vi "Inalfa SCU_LIN Message.vi"(0 "Sequence State in":T2, 1 "LIN Device":T4={"Master Frame(3C)"="MasterReq\nSPA3414_ConfigurationsCMAGeely_CEMCALYPSOSDB34XX0Cfg_LIN3_190709_", "Slave Frame(3D)"="SlaveResp\nSPA3414_ConfigurationsCMAGeely_CEMCALYPSOSDB34XX0Cfg_LIN3_190709_", "Request Schedule"="CEMLIN3DiagRequestSchedule\nSPA3414_ConfigurationsCMAGeely_CEMCALYPSOSDB34XX0Cfg_LIN3_190709_", "Response Schedule"="CEMLIN3DiagResponseSchedule\nSPA3414_ConfigurationsCMAGeely_CEMCALYPSOSDB34XX0Cfg_LIN3_190709_", "Frame Write SCU"="", "Frame Read SCU"="", "LIN Name"=""}, 3 "data bytes log in":string, 4 "Sequence State.Step Description":string, 5 "Sequence State.Step Data String":string, 6 "Mode type":string, 8 "NAD":u8) -> (7 "Software version":string[](array[string]), 10 "Calfile version":string[](array[string]), 11 "Hardware version":string[](array[string]), 12 "data bytes log out":string, 13 "Rx Message":u8[](array[numeric]) format="%02x", 14 "Response Good?":bool, 15 "Error Description":string, 17 "version type":T1(ring), 18 "Sequence State out":T2, 19 "Error No.":u16=132)   [LabVIEW 2018]
uses:
  LIN Device.ctl
  02.Type Def's/sequence state.ctl
  05.UserVI's/sequence/type defs/Sequence Info.ctl
  LIN show messages.ctl
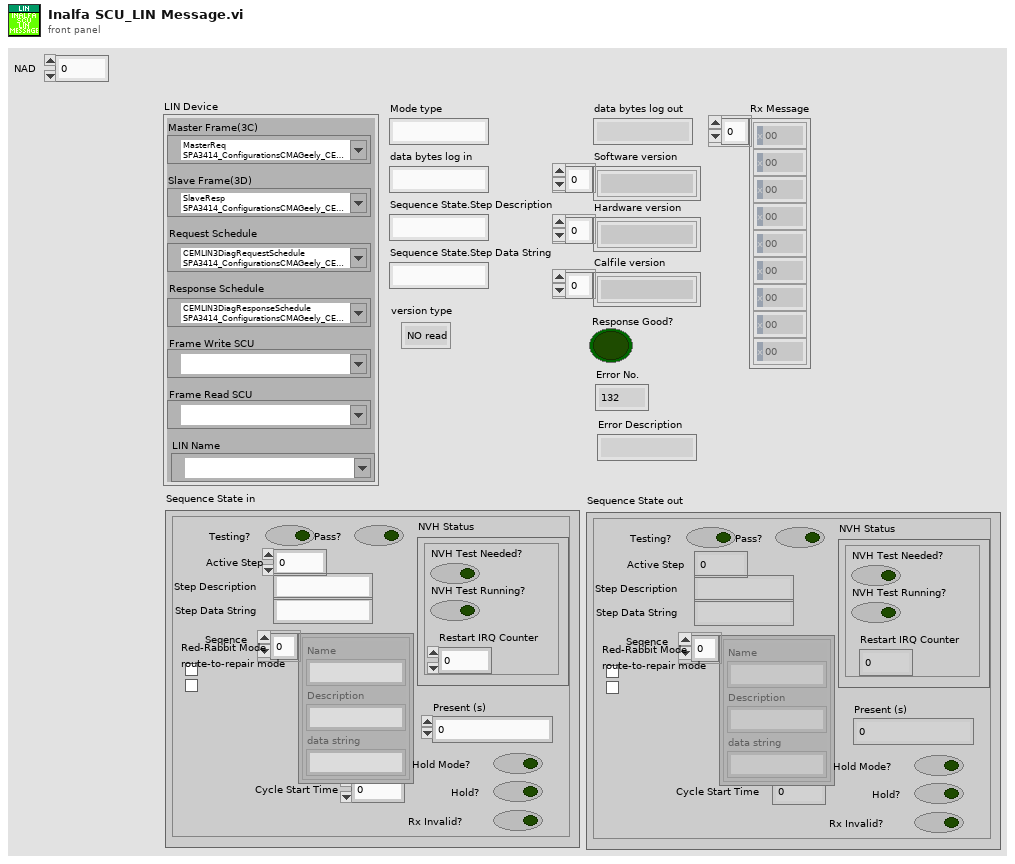
[diagram p1: front panel]
types:
  T1 = enum16{"NO read", "Softeware version", "Hardware version", "Calfile version"}
  T2 = typedef "sequence state.ctl" = cluster{"Step Description":string, "Cycle Start Time":u32, "Step Data String":string, "Pass?":bool, "Seqence":T3[], "Active Step":u8, "Testing?":bool, "Red-Rabbit Mode":bool, "route-to-repair mode":bool, "NVH Status":cluster{"Restart IRQ Counter":u8, "NVH Test Needed?":bool, "NVH Test Running?":bool}, "Present (s)":dbl, "Hold Mode?":bool, "Hold?":bool, "Rx Invalid?":bool}
  T3 = typedef "Sequence Info.ctl" = cluster{"Name":string, "Description":string, "data string":string}
  T4 = typedef "LIN Device.ctl" = cluster{"Master Frame(3C)":refnum<k21>, "Slave Frame(3D)":refnum<k21>, "Request Schedule":refnum<k21>, "Response Schedule":refnum<k21>, "Frame Write SCU":refnum<k21>, "Frame Read SCU":refnum<k21>, "LIN Name":refnum<k21>}
  T5 = typedef "LIN show messages.ctl" = cluster{"Slide Cycles":u16, "Vent Cycles":u16, "String":string, "Tx Bytes":u8[][], "Rx Bytes":u8[], "Only Tx1 Bytes":u8[][], "Go to Position":u16, "Check Glass Position":u16, "Checkgalss":bool, "Check Sunshade Position":u16, "Checksunshade":bool}
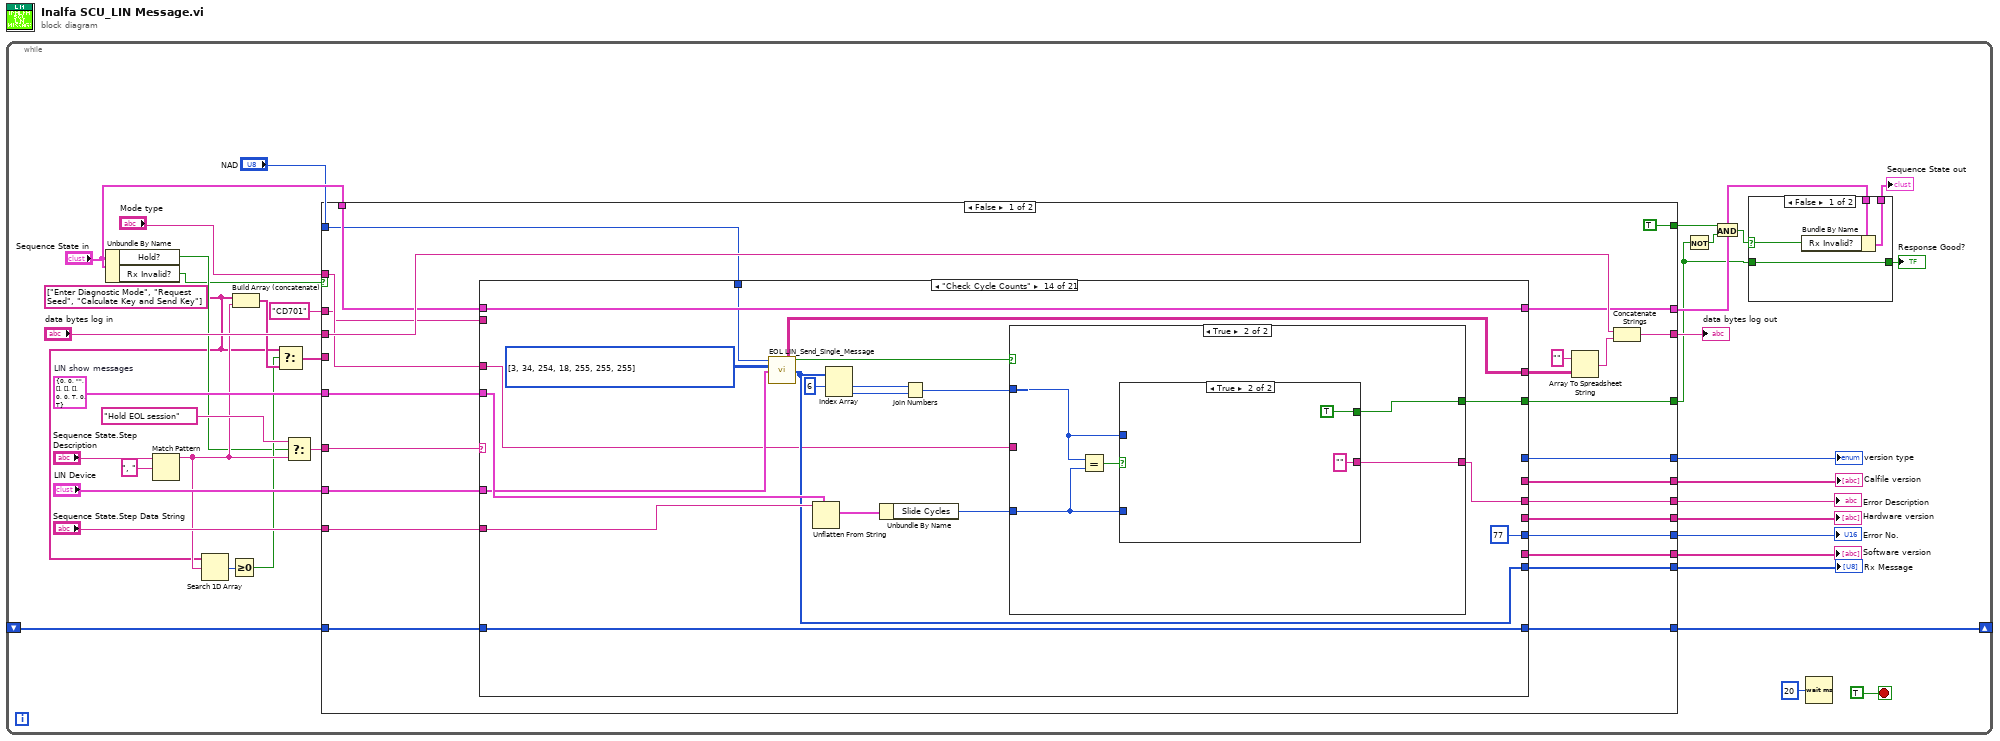
[diagram p0: block diagram]
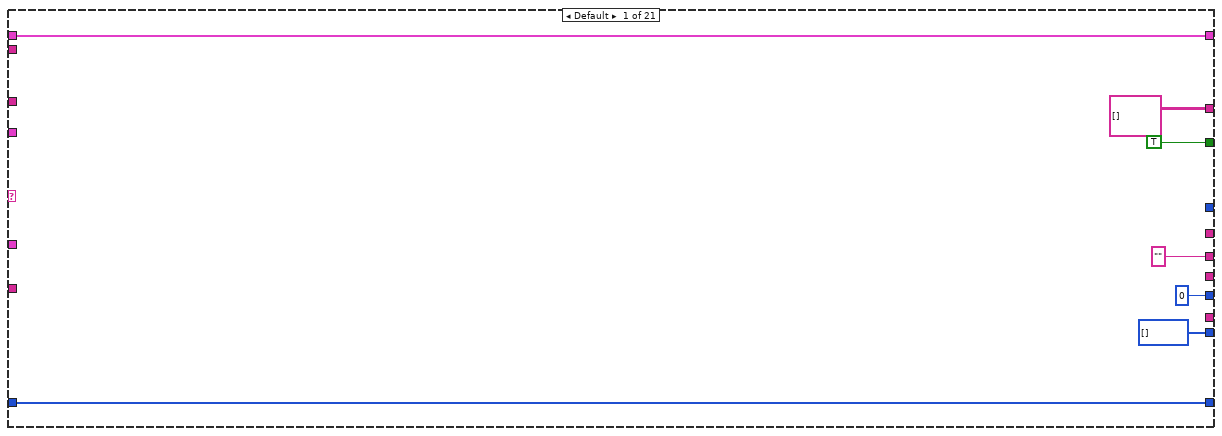
[diagram p2: hidden frame]
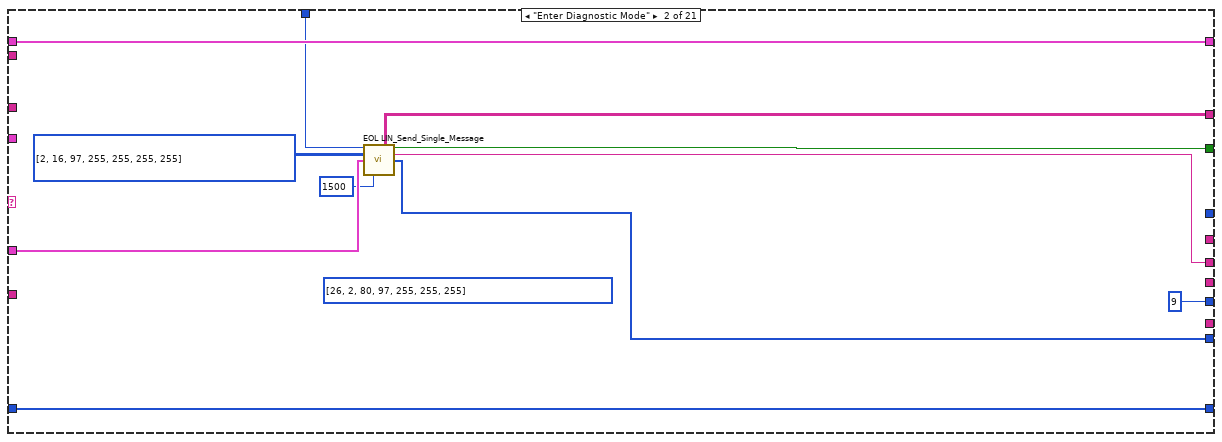
[diagram p3: hidden frame]
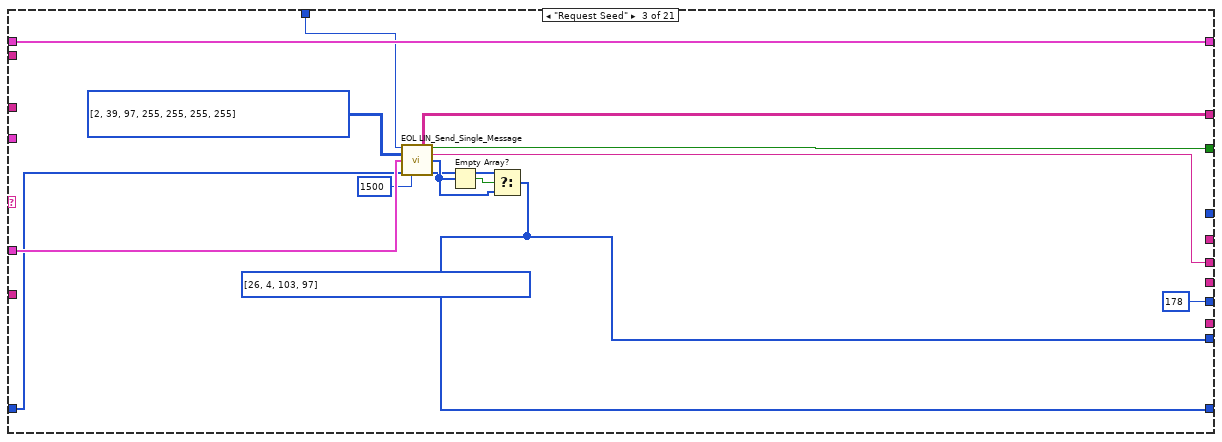
[diagram p4: hidden frame]
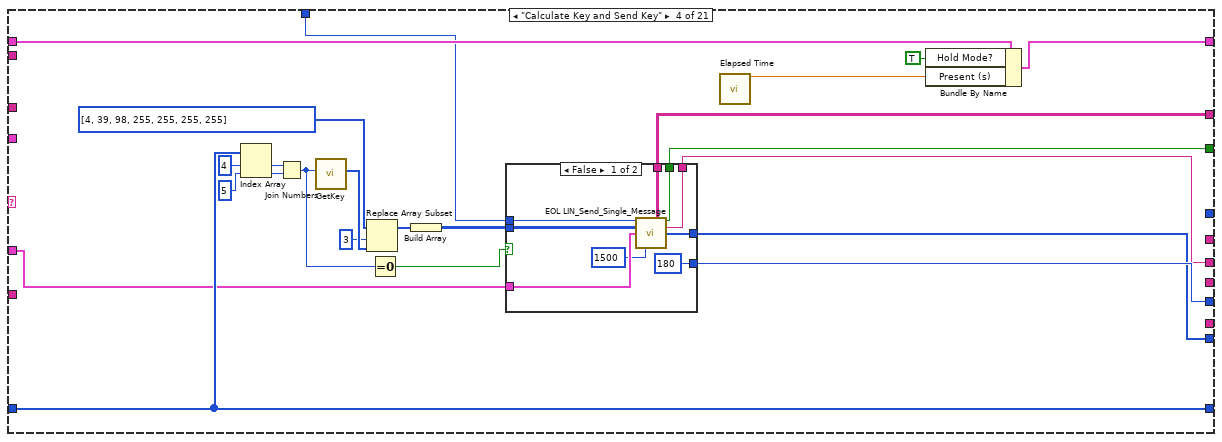
[diagram p5: hidden frame]
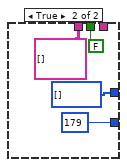
[diagram p6: hidden frame]
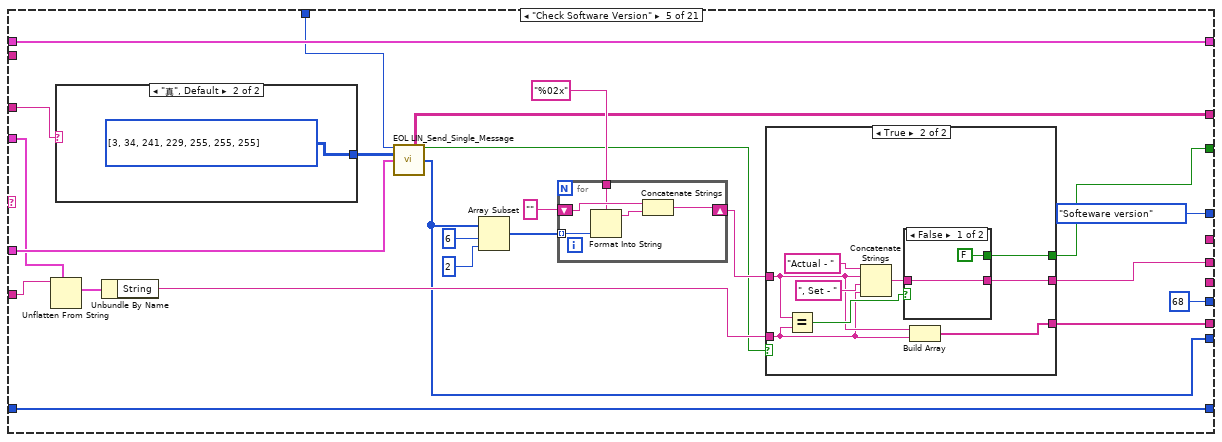
[diagram p7: hidden frame]
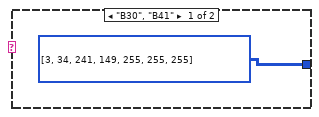
[diagram p8: hidden frame]
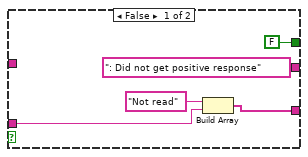
[diagram p9: hidden frame]
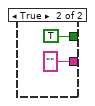
[diagram p10: hidden frame]
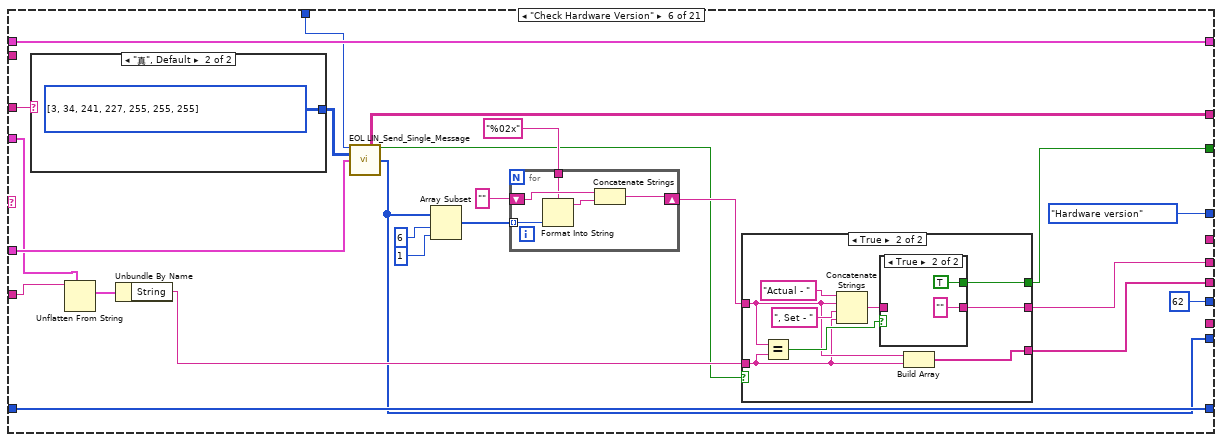
[diagram p11: hidden frame]
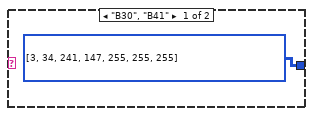
[diagram p12: hidden frame]
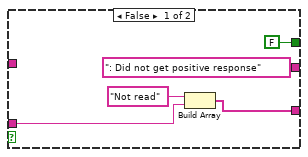
[diagram p13: hidden frame]
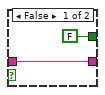
[diagram p14: hidden frame]
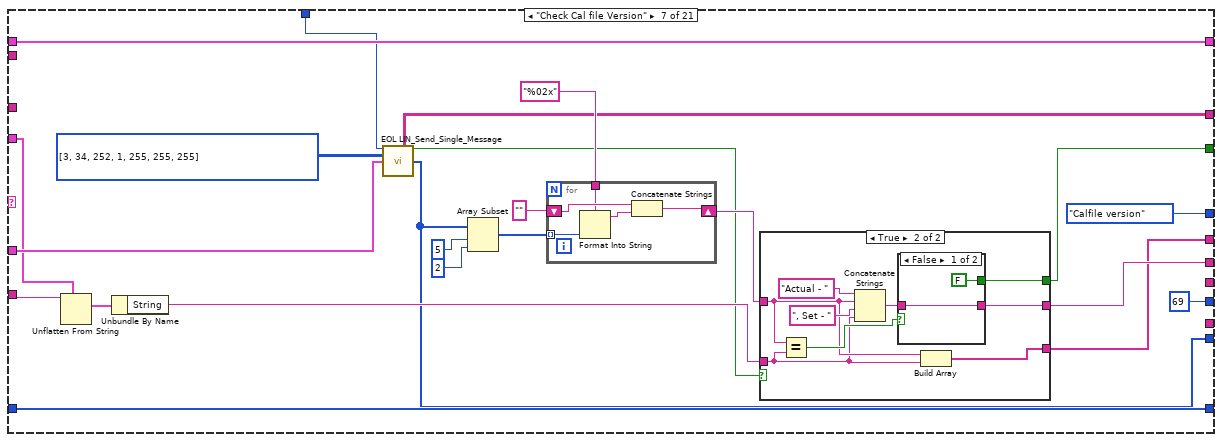
[diagram p15: hidden frame]
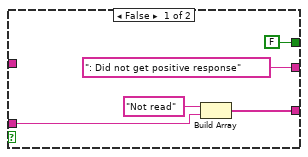
[diagram p16: hidden frame]
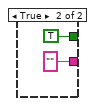
[diagram p17: hidden frame]
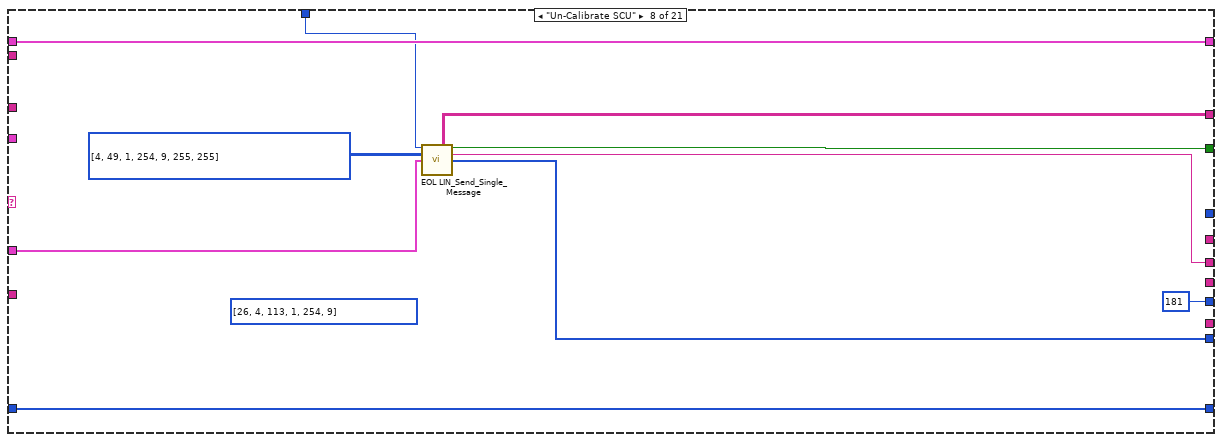
[diagram p18: hidden frame]
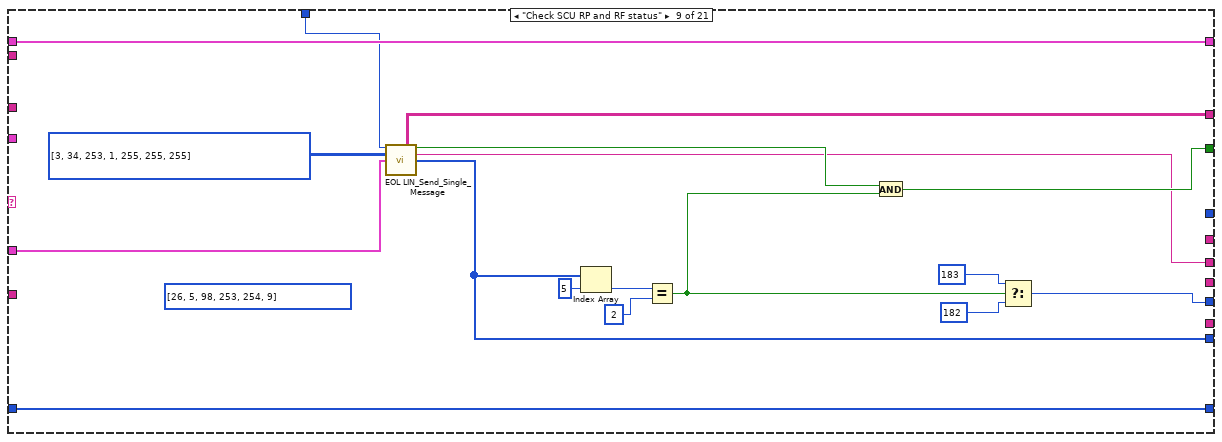
[diagram p19: hidden frame]
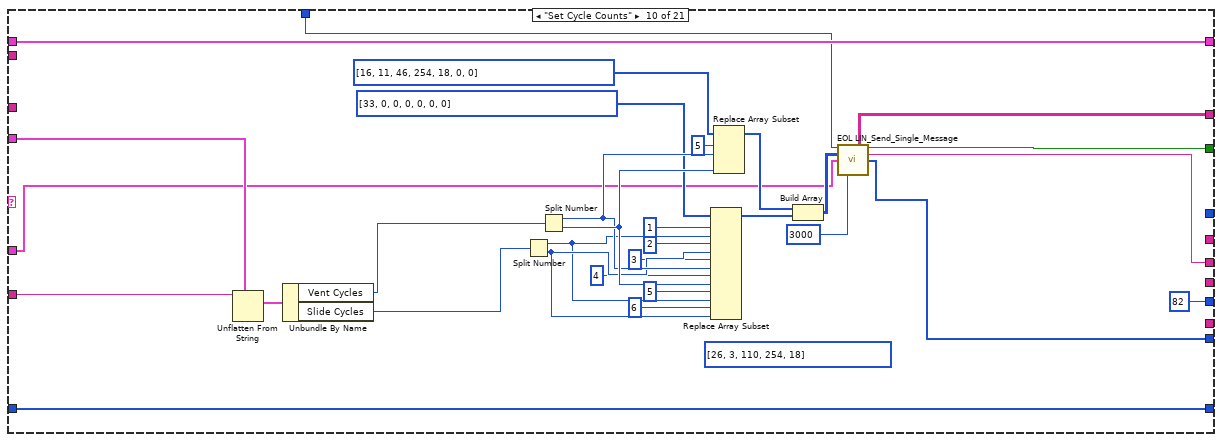
[diagram p20: hidden frame]
diagram:
  n1 = while {
    shift-right: [w33] -> _
    shift-left: _ -> [w32]
    stop <- TRUE stop-if-true
    w11 = string[] ["Enter Diagnostic Mode", "Request Seed", "Calculate Key and Send Key"]
    w36 = T5 {"Slide Cycles"=0, "Vent Cycles"=0, "String"="", "Tx Bytes"=[], "Rx Bytes"=[], "Only Tx1 Bytes"=[], "Go to Position"=0, "Check Glass Position"=0, "Checkgalss"=TRUE, "Check Sunshade Position"=0, "Checksunshade"=TRUE}  # LIN show messages
    n2 = Unbundle By Name("Sequence State in") -> ("Hold?"=w13:bool, "Rx Invalid?"=w12:bool)
    n3 = Match Pattern(string="Sequence State.Step Description", regular expression=", ") -> (before substring=w17:string)  [unwired: 1 in, 3 out]
    n4 = Search 1D Array(1D array=w11, element=w17) -> (index of element=w1:i32)  [unwired: 1 in]
    n5 = Greater Or Equal To 0?(x=w1) -> (x >= 0?=w14:bool)
    n6 = Build Array (concatenate)(w11, w17) -> (w16:string[])
    n7 = Select(t=w11, s=w14, f=w16) -> (s? t:f=w15:string[])
    n8 = Select(t="Hold EOL session", s=w13, f=w17) -> (s? t:f=w30:string)
    n9 = case shown="False" w12 {
      tunnel: "LIN Device" -> [w64 w636]
      tunnel: w36 -> [w63 w637]
      tunnel: [w62 w634] -> w35
      tunnel: [w61 w631] -> w33
      tunnel: w32 -> [w60 w623]
      tunnel: w30 -> [w59 w616]
      tunnel: [w45 w632] -> w20
      tunnel: [w58 w635] -> w3
      tunnel: [w56 w633] -> w26
      tunnel: "Sequence State.Step Data String" -> [w57 w626]
      tunnel: "data bytes log in" -> [w51 w630]
      tunnel: [w53 w629] -> w23
      tunnel: "Sequence State in" -> [w50 w628]
      tunnel: [w49 w627] -> w21
      tunnel: w15 -> [_ w625]
      tunnel: [TRUE FALSE] -> w19
      tunnel: "NAD" -> [w47 w622]
      tunnel: "Mode type" -> [w46 w621]
      tunnel: [w44 w618] -> w9
      tunnel: [w43 w619] -> w8
      tunnel: [w42 w620] -> w7
      tunnel: [w41 w617] -> w6
      tunnel: "CD701" -> [w40 w615]
      frame False {
        n10 = case shown="\"Check Cycle Counts\"" w59 {
          tunnel: w64 -> [_ w81 w92 w103 w154 w194 w245 w284 w301 w309 w343 w364 w394 w493 w528 w538 w546 w559 w576 w587 w610]
          tunnel: [string[][] [] ("TxRx Data") w80 w94 w107 w148 w203 w247 w283 w300 w315 w346 w368 w399 w496 w529 w539 w550 w563 w579 w601 w614] -> w52
          tunnel: [TRUE ("Response Good?") w76 w87 w105 w140 w189 w238 w279 w297 w307 w337 w367 w383 w486 w524 w534 w549 TRUE ("Response Good?") w570 w600 w613] -> w58
          tunnel: w57 -> [_ _ _ _ w146 w195 w243 _ _ w333 w357 w379 w401 w498 _ _ w551 w564 w580 w594 _]
          tunnel: w63 -> [_ _ _ _ w136 w184 w232 _ _ w312 w358 w380 w400 w497 _ _ w552 w565 w581 w595 _]
          tunnel: ["" ("spreadsheet string") w75 w86 w100 w143 w197 w240 w278 w291 w306 w338 w362 w382 w485 w523 w533 w543 w556 w569 w586 w606] -> w62
          tunnel: [u16 0 ("Error No.") u16 9 ("Error No.") u16 178 ("Error No.") w104 u16 68 ("Error No.") u16 62 ("Error No.") u16 69 ("Error No.") u16 181 ("Error No.") w294 u16 82 ("Error No.") u16 184 ("Error No.") u16 185 ("Error No.") u16 20 ("Error No.") u16 77 ("Error No.") u16 55 ("Error No.") u16 55 ("Error No.") u16 56 ("Error No.") u16 0 ("Error No.") u16 56 ("Error No.") u16 186 ("Error No.") u16 187 ("Error No.")] -> w56
          tunnel: [w69 w78 w89 w106 w142 w191 w239 w282 w299 w311 w345 w366 w396 w495 w527 w537 w548 w561 w578 w599 w612] -> w61
          tunnel: w60 -> [w69 w78 w88 w106 w142 w191 w239 w282 w299 w311 w345 w366 w396 w495 w527 w537 w548 w561 w578 w599 w612]
          tunnel: [u8[] [] ("Rx Message") w77 w89 w102 w138 w187 w235 w280 w292 w308 w342 w363 w393 w492 w525 w535 w545 w558 w574 w597 w609] -> w45
          tunnel: w50 -> [w65 w74 w85 w98 w137 w186 w234 w277 w290 w305 w341 w361 w392 w491 w522 w532 w542 w555 w568 w585 w605]
          tunnel: [w65 w74 w85 w97 w137 w186 w234 w277 w290 w305 w341 w361 w392 w491 w522 w532 w542 w555 w568 w585 w604] -> w49
          tunnel: w47 -> [_ w73 w84 w96 w135 w185 w233 w276 w289 w304 w340 w360 w391 w490 w521 w531 w541 w554 w567 w584 w603]
          tunnel: w46 -> [_ _ _ _ w132 w183 _ _ _ _ w336 _ w381 w484 _ _ _ _ _ _ _]
          tunnel: [_ _ _ _ w134 _ _ _ _ _ _ _ _ _ _ _ _ _ _ _ _] -> w44
          tunnel: [_ _ _ _ _ w182 _ _ _ _ _ _ _ _ _ _ _ _ _ _ _] -> w43
          tunnel: [_ _ _ _ _ _ w231 _ _ _ _ _ _ _ _ _ _ _ _ _ _] -> w42
          tunnel: [_ _ _ _ T1."Softeware version" ("version type") T1."Hardware version" ("version type") T1."Calfile version" ("version type") _ _ _ _ _ _ _ _ _ _ _ _ _ _] -> w41
          tunnel: w40 -> [_ _ _ _ _ _ _ _ _ _ w335 _ _ _ _ _ _ _ _ _ _]
          frame Default {
          }
          frame "Enter Diagnostic Mode" {
            (unwired) u8[] [26, 2, 80, 97, 255, 255, 255]
            n11 = call "EOL LIN_Send_Single_Message.vi"("NAD"=w73, "Tx Msg"=u8[][] [[2, 16, 97, 255, 255, 255, 255]], "LIN Device"=w81, "Msg Wait Time"=u32 1500) -> ("TxRx Data"=w80:string[][], "Response Good?"=w76:bool, "spreadsheet string"=w75:string, "Rx Msg"=w77:u8[])  [unwired: 7 in, 1 out]
          }
          frame "Request Seed" {
            (unwired) u8[] [26, 4, 103, 97]
            n12 = call "EOL LIN_Send_Single_Message.vi"("NAD"=w84, "Tx Msg"=u8[][] [[2, 39, 97, 255, 255, 255, 255]], "LIN Device"=w92, "Msg Wait Time"=u32 1500) -> ("TxRx Data"=w94:string[][], "Response Good?"=w87:bool, "spreadsheet string"=w86:string, "Rx Msg"=w90:u8[])  [unwired: 7 in, 1 out]
            n13 = Empty Array?(array=w90) -> (empty?=w91:bool)
            n14 = Select(t=w88, s=w91, f=w90) -> (s? t:f=w89:u8[])
          }
          frame "Calculate Key and Send Key" {
            n15 = Index Array(array=w106, index #1=4 ("index"), index #2=5 ("index")) -> (element #1=w116:u8, element #2=w115:u8)
            n16 = Join Numbers(hi=w116, lo=w115) -> ((hi.lo)=w110:u16)
            n17 = call "GetKey.vi"("x"=w110) -> ("KEY"=w114:u8[])  [unwired: 10 in]
            n18 = Replace Array Subset(array=u8[] [4, 39, 98, 255, 255, 255, 255], new element=w114, index=3) -> (w111:u8[])
            n19 = Equal To 0?(x=w110) -> (x = 0?=w108:bool)
            n20 = Build Array(w111) -> (w109:u8[][])
            n21 = case shown="False" w108 {
              tunnel: w109 -> [w127 _]
              tunnel: [w126 string[][] [] ("TxRx Data")] -> w107
              tunnel: [w125 FALSE ("Response Good?")] -> w105
              tunnel: [w124 _] -> w100
              tunnel: [u16 180 ("Error No.") u16 179 ("Error No.")] -> w104
              tunnel: w103 -> [w122 _]
              tunnel: [w121 u8[] [] ("Rx Message")] -> w102
              tunnel: w96 -> [w120 _]
              frame False {
                n22 = call "EOL LIN_Send_Single_Message.vi"("NAD"=w120, "Tx Msg"=w127, "LIN Device"=w122, "Msg Wait Time"=u32 1500) -> ("TxRx Data"=w126:string[][], "Response Good?"=w125:bool, "spreadsheet string"=w124:string, "Rx Msg"=w121:u8[])  [unwired: 7 in, 1 out]
              }
              frame True {
              }
            }
            n23 = call "Elapsed Time"() -> ("Present (s)"=w101:dbl)  [unwired: 12 in, 7 out]
            n24 = Bundle By Name(cluster=w98, "Hold Mode?"=TRUE, "Present (s)"=w101) -> (w97:T2)
          }
          frame "Check Software Version" {
            n25 = Unflatten From String(type=w136, binary string=w146) -> (value=w147:T5)  [unwired: 3 in, 2 out]
            n26 = case shown="\"真\", Default" w132 {
              tunnel: [u8[][] [[3, 34, 241, 149, 255, 255, 255]] u8[][] [[3, 34, 241, 229, 255, 255, 255]]] -> w155
              frame "B30", "B41" {
              }
              frame "真", Default {
              }
            }
            n27 = Unbundle By Name(w147) -> ("String"=w144:string)
            n28 = call "EOL LIN_Send_Single_Message.vi"("NAD"=w135, "Tx Msg"=w155, "LIN Device"=w154) -> ("TxRx Data"=w148:string[][], "Response Good?"=w141:bool, "Rx Msg"=w138:u8[])  [unwired: 8 in, 2 out]
            n29 = Array Subset(array=w138, index=6, length=2) -> (w153:u8[])
            n30 = for {
              tunnel: w153 -> [w176] mode=indexing
              shift-right: [w179] -> w145
              shift-left: "" -> [w178]
              tunnel: "%02x" ("format string") -> [w177]
              n31 = Format Into String(format string=w177, w176) -> (resulting string=w180:string)  [unwired: 2 in, 1 out]
              n32 = Concatenate Strings(w178, w180) -> (w179:string)
            }
            n33 = case shown="True" w141 {
              tunnel: w145 -> [_ w165]
              tunnel: w144 -> [w159 w164]
              tunnel: [FALSE w167] -> w140
              tunnel: [w158 w163] -> w134
              tunnel: [": Did not get positive response" ("Error Description") w166] -> w143
              frame False {
                n34 = Build Array("Not read" ("Constant level"), w159) -> (w158:string[])
              }
              frame True {
                n35 = Equal?(x=w165, y=w164) -> (x = y?=w168:bool)
                n36 = Concatenate Strings("Actual - " ("string"), w165, ", Set - " ("string"), w164) -> (w169:string)
                n37 = case shown="False" w168 {
                  tunnel: w169 -> [w172 _]
                  tunnel: [FALSE TRUE] -> w167
                  tunnel: [w172 ""] -> w166
                  frame False {
                  }
                  frame True {
                  }
                }
                n38 = Build Array(w165, w164) -> (w163:string[])
              }
            }
          }
          frame "Check Hardware Version" {
            n39 = case shown="\"真\", Default" w183 {
              tunnel: [u8[][] [[3, 34, 241, 147, 255, 255, 255]] u8[][] [[3, 34, 241, 227, 255, 255, 255]]] -> w204
              frame "B30", "B41" {
              }
              frame "真", Default {
              }
            }
            n40 = Unflatten From String(type=w184, binary string=w195) -> (value=w196:T5)  [unwired: 3 in, 2 out]
            n41 = Unbundle By Name(w196) -> ("String"=w193:string)
            n42 = call "EOL LIN_Send_Single_Message.vi"("NAD"=w185, "Tx Msg"=w204, "LIN Device"=w194) -> ("TxRx Data"=w203:string[][], "Response Good?"=w190:bool, "Rx Msg"=w187:u8[])  [unwired: 8 in, 2 out]
            n43 = Array Subset(array=w187, index=6, length=1) -> (w202:u8[])
            n44 = for {
              tunnel: w202 -> [w225] mode=indexing
              shift-right: [w228] -> w192
              shift-left: "" -> [w227]
              tunnel: "%02x" ("format string") -> [w226]
              n45 = Format Into String(format string=w226, w225) -> (resulting string=w229:string)  [unwired: 2 in, 1 out]
              n46 = Concatenate Strings(w227, w229) -> (w228:string)
            }
            n47 = case shown="True" w190 {
              tunnel: w192 -> [_ w214]
              tunnel: w193 -> [w208 w213]
              tunnel: [FALSE w216] -> w189
              tunnel: [w207 w212] -> w182
              tunnel: [": Did not get positive response" ("Error Description") w215] -> w197
              frame False {
                n48 = Build Array("Not read" ("Constant level"), w208) -> (w207:string[])
              }
              frame True {
                n49 = Equal?(x=w214, y=w213) -> (x = y?=w217:bool)
                n50 = Concatenate Strings("Actual - " ("string"), w214, ", Set - " ("string"), w213) -> (w218:string)
                n51 = case shown="True" w217 {
                  tunnel: w218 -> [w221 _]
                  tunnel: [FALSE TRUE] -> w216
                  tunnel: [w221 ""] -> w215
                  frame False {
                  }
                  frame True {
                  }
                }
                n52 = Build Array(w214, w213) -> (w212:string[])
              }
            }
          }
          frame "Check Cal file Version" {
            n53 = Unflatten From String(type=w232, binary string=w243) -> (value=w244:T5)  [unwired: 3 in, 2 out]
            n54 = Unbundle By Name(w244) -> ("String"=w242:string)
            n55 = call "EOL LIN_Send_Single_Message.vi"("NAD"=w233, "Tx Msg"=u8[][] [[3, 34, 252, 1, 255, 255, 255]], "LIN Device"=w245) -> ("TxRx Data"=w247:string[][], "Response Good?"=w237:bool, "Rx Msg"=w235:u8[])  [unwired: 8 in, 2 out]
            n56 = Array Subset(array=w235, index=5, length=2) -> (w252:u8[])
            n57 = for {
              tunnel: w252 -> [w271] mode=indexing
              shift-right: [w274] -> w241
              shift-left: "" -> [w273]
              tunnel: "%02x" ("format string") -> [w272]
              n58 = Format Into String(format string=w272, w271) -> (resulting string=w275:string)  [unwired: 2 in, 1 out]
              n59 = Concatenate Strings(w273, w275) -> (w274:string)
            }
            n60 = case shown="True" w237 {
              tunnel: w241 -> [_ w260]
              tunnel: w242 -> [w254 w259]
              tunnel: [FALSE w262] -> w238
              tunnel: [w253 w258] -> w231
              tunnel: [": Did not get positive response" ("Error Description") w261] -> w240
              frame False {
                n61 = Build Array("Not read" ("Constant level"), w254) -> (w253:string[])
              }
              frame True {
                n62 = Equal?(x=w260, y=w259) -> (x = y?=w263:bool)
                n63 = Concatenate Strings("Actual - " ("string"), w260, ", Set - " ("string"), w259) -> (w264:string)
                n64 = case shown="False" w263 {
                  tunnel: w264 -> [w267 _]
                  tunnel: [FALSE TRUE] -> w262
                  tunnel: [w267 ""] -> w261
                  frame False {
                  }
                  frame True {
                  }
                }
                n65 = Build Array(w260, w259) -> (w258:string[])
              }
            }
          }
          frame "Un-Calibrate SCU" {
            (unwired) u8[] [26, 4, 113, 1, 254, 9]
            n66 = call "EOL LIN_Send_Single_Message.vi"("NAD"=w276, "Tx Msg"=u8[][] [[4, 49, 1, 254, 9, 255, 255]], "LIN Device"=w284) -> ("TxRx Data"=w283:string[][], "Response Good?"=w279:bool, "spreadsheet string"=w278:string, "Rx Msg"=w280:u8[])  [unwired: 8 in, 1 out]
          }
          frame "Check SCU RP and RF status" {
            (unwired) u8[] [26, 5, 98, 253, 254, 9]
            n67 = call "EOL LIN_Send_Single_Message.vi"("NAD"=w289, "Tx Msg"=u8[][] [[3, 34, 253, 1, 255, 255, 255]], "LIN Device"=w301) -> ("TxRx Data"=w300:string[][], "Response Good?"=w298:bool, "spreadsheet string"=w291:string, "Rx Msg"=w292:u8[])  [unwired: 8 in, 1 out]
            n68 = Index Array(array=w292, index=5) -> (element=w287:u8)
            n69 = Equal?(x=w287, y=u8 2 ("element")) -> (x = y?=w286:bool)
            n70 = And(x=w298, y=w286) -> (x .and. y?=w297:bool)
            n71 = Select(t=u16 183 ("Error No."), s=w286, f=u16 182 ("Error No.")) -> (s? t:f=w294:u16)
          }
          frame "Set Cycle Counts" {
            (unwired) u8[] [26, 3, 110, 254, 18]
            n72 = Unflatten From String(type=w312, binary string=w333) -> (value=w332:T5)  [unwired: 3 in, 2 out]
            n73 = Unbundle By Name(w332) -> ("Vent Cycles"=w314:u16, "Slide Cycles"=w313:u16)
            n74 = Split Number(x=w313) -> (hi(x)=w326:u8, lo(x)=w327:u8)
            n75 = Split Number(x=w314) -> (hi(x)=w328:u8, lo(x)=w329:u8)
            n76 = Replace Array Subset(array=u8[] [33, 0, 0, 0, 0, 0, 0] ("Frame payloads to queue"), new element #1=w326, index #1=1 ("索引"), new element #2=w327, index #2=2 ("索引"), new element #3=w328, index #3=3 ("索引"), new element #4=w329, index #4=4 ("索引"), new element #5=w326, index #5=5 ("索引"), new element #6=w327, index #6=6 ("索引")) -> (w331:u8[])
            n77 = Replace Array Subset(array=u8[] [16, 11, 46, 254, 18, 0, 0] ("Frame payloads to queue"), new element #1=w328, index #1=5 ("索引"), new element #2=w329) -> (w330:u8[])  [unwired: 1 in]
            n78 = Build Array(w330, w331) -> (w316:u8[][])
            n79 = call "EOL LIN_Send_Single_Message.vi"("NAD"=w304, "Tx Msg"=w316, "LIN Device"=w309, "Msg Wait Time"=u32 3000) -> ("TxRx Data"=w315:string[][], "Response Good?"=w307:bool, "spreadsheet string"=w306:string, "Rx Msg"=w308:u8[])  [unwired: 7 in, 1 out]
          }
          frame "Go to position glass" {
            n80 = Equal?(x=w335, y=w336) -> (x = y?=w334:bool)
            n81 = Unflatten From String(type=w358, binary string=w357) -> (value=w356:T5)  [unwired: 3 in, 2 out]
            n82 = Unbundle By Name(w356) -> ("Go to Position"=w355:u16)
            n83 = Split Number(x=w355) -> (hi(x)=w352:u8, lo(x)=w351:u8)
            n84 = Replace Array Subset(array=u8[] [33, 0, 0, 0, 0, 255, 255], new element #1=w352, index #1=1 ("index"), new element #2=w351, index #2=2 ("index")) -> (w349:u8[])
            n85 = Build Array(u8[] [16, 9, 49, 1, 253, 4, 1], w349) -> (w347:u8[][])
            n86 = call "EOL LIN_Send_Single_Message.vi"("NAD"=w340, "CD701 position"=w334, "Tx Msg"=w347, "LIN Device"=w343, "Msg Wait Time"=u32 3000) -> ("TxRx Data"=w346:string[][], "Response Good?"=w337:bool, "spreadsheet string"=w338:string, "Rx Msg"=w342:u8[])  [unwired: 6 in, 1 out]
          }
          frame "Go to position sunshade" {
            n87 = Unflatten From String(type=w380, binary string=w379) -> (value=w378:T5)  [unwired: 3 in, 2 out]
            n88 = Unbundle By Name(w378) -> ("Go to Position"=w377:u16)
            n89 = Split Number(x=w377) -> (hi(x)=w374:u8, lo(x)=w373:u8)
            n90 = Replace Array Subset(array=u8[] [33, 0, 0, 0, 0, 255, 255], new element #1=w374, index #1=3 ("index"), new element #2=w373, index #2=4 ("index")) -> (w371:u8[])
            n91 = Build Array(u8[] [16, 9, 49, 1, 253, 4, 2], w371) -> (w369:u8[][])
            n92 = call "EOL LIN_Send_Single_Message.vi"("NAD"=w360, "Tx Msg"=w369, "LIN Device"=w364, "Msg Wait Time"=u32 3000) -> ("TxRx Data"=w368:string[][], "Response Good?"=w367:bool, "spreadsheet string"=w362:string, "Rx Msg"=w363:u8[])  [unwired: 7 in, 1 out]
          }
          frame "Check hall position glass and sunshade" {
            n93 = call "EOL LIN_Send_Single_Message.vi"("NAD"=w391, "Tx Msg"=u8[][] [[3, 34, 253, 2, 255, 255, 255]], "LIN Device"=w394) -> ("TxRx Data"=w399:string[][], "Response Good?"=w390:bool, "Rx Msg"=w393:u8[])  [unwired: 8 in, 2 out]
            n94 = Unflatten From String(type=w400, binary string=w401) -> (value=w402:T5)  [unwired: 3 in, 2 out]
            n95 = Index Array(array=w393, index #1=6 ("index"), index #3=8 ("index")) -> (element #1=w405:u8, element #2=w404:u8, element #3=w398:u8, element #4=w397:u8)  [unwired: 2 in]
            n96 = Unbundle By Name(w402) -> ("Check Glass Position"=w387:u16, "Checkgalss"=w386:bool, "Check Sunshade Position"=w385:u16, "Checksunshade"=w384:bool)
            n97 = Join Numbers(hi=w405, lo=w404) -> ((hi.lo)=w389:u16)
            n98 = Join Numbers(hi=w398, lo=w397) -> ((hi.lo)=w388:u16)
            n99 = case shown="True" w390 {
              tunnel: w389 -> [_ w412]
              tunnel: w387 -> [_ w413]
              tunnel: ["Could not get reponse during Check Motor Hall Position" ("Error Description") w414] -> w382
              tunnel: [FALSE w417] -> w383
              tunnel: w386 -> [_ w416]
              tunnel: w384 -> [_ w415]
              tunnel: w388 -> [_ w411]
              tunnel: w385 -> [_ w418]
              tunnel: w381 -> [_ w410]
              frame False {
              }
              frame True {
                n100 = case shown="\"CD701\"" w410 {
                  tunnel: w418 -> [_ w464]
                  tunnel: [w419 w461] -> w417
                  tunnel: w416 -> [w423 w457]
                  tunnel: w415 -> [_ w453]
                  tunnel: [w422 w449] -> w414
                  tunnel: w413 -> [w421 w448]
                  tunnel: w412 -> [w420 w444]
                  tunnel: w411 -> [_ w443]
                  frame "CD701" {
                    n101 = Not Equal To 0?(x=w420) -> (x != 0?=w433:bool)
                    n102 = Add(x=u16 40, y=w421) -> (x+y=w438:u16)
                    n103 = Subtract(x=w421, y=u16 40) -> (x-y=w435:u16)
                    n104 = In Range and Coerce(upper limit=w438, x=w420, lower limit=w435) -> (In Range?=w432:bool)  [unwired: 1 out]
                    n105 = And(x=w433, y=w432) -> (x .and. y?=w431:bool)
                    n106 = Select(t=w431, s=w423, f=TRUE) -> (s? t:f=w419:bool)
                    n107 = Format Into String(initial string=", Max Lt ", w438) -> (resulting string=w437:string)  [unwired: 2 in, 1 out]
                    n108 = Format Into String(initial string=", Min Lt ", w435) -> (resulting string=w436:string)  [unwired: 2 in, 1 out]
                    n109 = Format Into String(initial string="Glass Actual  " ("string"), w420) -> (resulting string=w439:string)  [unwired: 2 in, 1 out]
                    n110 = Concatenate Strings(w439, w437, w436) -> (w434:string)
                    n111 = Select(t=w434, s=w423, f="") -> (s? t:f=w422:string)
                  }
                  frame "NU2", Default {
                    n112 = Not Equal To 0?(x=w444) -> (x != 0?=w447:bool)
                    n113 = Not Equal To 0?(x=w443) -> (x != 0?=w442:bool)
                    n114 = Add(x=u16 40, y=w448) -> (x+y=w479:u16)
                    n115 = Subtract(x=w448, y=u16 40) -> (x-y=w475:u16)
                    n116 = Add(x=u16 20, y=w464) -> (x+y=w468:u16)
                    n117 = Subtract(x=w464, y=u16 20) -> (x-y=w470:u16)
                    n118 = In Range and Coerce(upper limit=w479, x=w444, lower limit=w475) -> (In Range?=w446:bool)  [unwired: 1 out]
                    n119 = In Range and Coerce(upper limit=w468, x=w443, lower limit=w470) -> (In Range?=w441:bool)  [unwired: 1 out]
                    n120 = And(x=w447, y=w446) -> (x .and. y?=w445:bool)
                    n121 = And(x=w442, y=w441) -> (x .and. y?=w440:bool)
                    n122 = Select(t=w445, s=w457, f=TRUE) -> (s? t:f=w463:bool)
                    n123 = Select(t=w440, s=w453, f=TRUE) -> (s? t:f=w462:bool)
                    n124 = And(x=w463, y=w462) -> (x .and. y?=w461:bool)
                    n125 = Format Into String(initial string="Glass Actual  " ("string"), w444) -> (resulting string=w483:string)  [unwired: 2 in, 1 out]
                    n126 = Format Into String(initial string=", Max Lt ", w479) -> (resulting string=w477:string)  [unwired: 2 in, 1 out]
                    n127 = Format Into String(initial string=", Min Lt ", w475) -> (resulting string=w476:string)  [unwired: 2 in, 1 out]
                    n128 = Format Into String(initial string="。Sunshade Actual  " ("string"), w443) -> (resulting string=w460:string)  [unwired: 2 in, 1 out]
                    n129 = Format Into String(initial string=", Max Lt ", w468) -> (resulting string=w459:string)  [unwired: 2 in, 1 out]
                    n130 = Format Into String(initial string=", Min Lt ", w470) -> (resulting string=w458:string)  [unwired: 2 in, 1 out]
                    n131 = Concatenate Strings(w460, w459, w458) -> (w452:string)
                    n132 = Concatenate Strings(w483, w477, w476) -> (w456:string)
                    n133 = Select(t=w456, s=w457, f="") -> (s? t:f=w451:string)
                    n134 = Select(t=w452, s=w453, f="") -> (s? t:f=w450:string)
                    n135 = Concatenate Strings(w451, w450) -> (w449:string)
                  }
                }
              }
            }
          }
          frame "Check Cycle Counts" {
            n136 = call "EOL LIN_Send_Single_Message.vi"("NAD"=w490, "Tx Msg"=u8[][] [[3, 34, 254, 18, 255, 255, 255]], "LIN Device"=w493) -> ("TxRx Data"=w496:string[][], "Response Good?"=w489:bool, "Rx Msg"=w492:u8[])  [unwired: 8 in, 2 out]
            n137 = Unflatten From String(type=w497, binary string=w498) -> (value=w499:T5)  [unwired: 3 in, 2 out]
            n138 = Index Array(array=w492, index #1=6 ("index")) -> (element #1=w501:u8, element #2=w500:u8)  [unwired: 1 in]
            n139 = Unbundle By Name(w499) -> ("Slide Cycles"=w487:u16)
            n140 = Join Numbers(hi=w501, lo=w500) -> ((hi.lo)=w488:u16)
            n141 = case shown="True" w489 {
              tunnel: w488 -> [_ w509]
              tunnel: w487 -> [_ w508]
              tunnel: ["Could not get reponse during Check Cycle Counts" ("Error Description") w510] -> w485
              tunnel: [FALSE w506] -> w486
              tunnel: w484 -> [_ _]
              frame False {
              }
              frame True {
                n142 = Equal?(x=w509, y=w508) -> (x = y?=w507:bool)
                n143 = case shown="True" w507 {
                  tunnel: [w514 ""] -> w510
                  tunnel: w509 -> [w513 _]
                  tunnel: w508 -> [w512 _]
                  tunnel: [FALSE TRUE] -> w506
                  frame False {
                    n144 = Format Into String(initial string=", Set - ", w512) -> (resulting string=w517:string)  [unwired: 2 in, 1 out]
                    n145 = Format Into String(initial string="Slide Cycle Actual - " ("string"), w513) -> (resulting string=w518:string)  [unwired: 2 in, 1 out]
                    n146 = Concatenate Strings(w518, w517) -> (w514:string)
                  }
                  frame True {
                  }
                }
              }
            }
          }
          frame "Clear DTC" {
            (unwired) u8[] [26, 1, 84]
            n147 = call "EOL LIN_Send_Single_Message.vi"("NAD"=w521, "Tx Msg"=u8[][] [[4, 20, 255, 255, 255, 255, 255]], "LIN Device"=w528) -> ("TxRx Data"=w529:string[][], "Response Good?"=w524:bool, "spreadsheet string"=w523:string, "Rx Msg"=w525:u8[])  [unwired: 8 in, 1 out]
          }
          frame "Check DTC" {
            n148 = call "EOL LIN_Send_Single_Message.vi"("NAD"=w531, "Tx Msg"=u8[][] [[3, 34, 254, 42, 255, 255, 255]], "LIN Device"=w538) -> ("TxRx Data"=w539:string[][], "Response Good?"=w534:bool, "spreadsheet string"=w533:string, "Rx Msg"=w535:u8[])  [unwired: 8 in, 1 out]
          }
          frame "Send Single Message" {
            n149 = Unflatten From String(type=w552, binary string=w551) -> (value=w553:T5)  [unwired: 3 in, 2 out]
            n150 = Unbundle By Name(w553) -> ("Only Tx1 Bytes"=w544:u8[][])
            n151 = call "EOL LIN_Send_Single_Message.vi"("NAD"=w541, "Tx Msg"=w544, "LIN Device"=w546) -> ("TxRx Data"=w550:string[][], "Response Good?"=w549:bool, "spreadsheet string"=w543:string, "Rx Msg"=w545:u8[])  [unwired: 8 in, 1 out]
          }
          frame "Send Single Message With Out Rx" {
            n152 = Unflatten From String(type=w565, binary string=w564) -> (value=w566:T5)  [unwired: 3 in, 2 out]
            n153 = Unbundle By Name(w566) -> ("Only Tx1 Bytes"=w557:u8[][])
            n154 = call "EOL LIN_Send_Single_Message.vi"("NAD"=w554, "Tx Msg"=w557, "LIN Device"=w559) -> ("TxRx Data"=w563:string[][], "spreadsheet string"=w556:string, "Rx Msg"=w558:u8[])  [unwired: 8 in, 2 out]
          }
          frame "Send Single Message With Response" {
            n155 = Unflatten From String(type=w581, binary string=w580) -> (value=w582:T5)  [unwired: 3 in, 2 out]
            n156 = Unbundle By Name(w582) -> ("Tx Bytes"=w575:u8[][], "Rx Bytes"=w573:u8[])
            n157 = call "EOL LIN_Send_Single_Message.vi"("NAD"=w567, "Tx Msg"=w575, "LIN Device"=w576) -> ("TxRx Data"=w579:string[][], "Response Good?"=w572:bool, "spreadsheet string"=w569:string, "Rx Msg"=w574:u8[])  [unwired: 8 in, 1 out]
            n158 = call "Check Response Bytes.vi"("Data Bytes"=w573, "Response Bytes"=w574) -> ("Pass?"=w571:bool)  [unwired: 9 in]
            n159 = And(x=w572, y=w571) -> (x .and. y?=w570:bool)
          }
          frame "Inalfa SCU Teach" {
            (unwired) u8[][] [[5, 49, 1, 240, 0, 0, 255]]
            n160 = Unflatten From String(type=w595, binary string=w594) -> (value=w596:T5)  [unwired: 3 in, 2 out]
            n161 = Unbundle By Name(w596) -> ("String"=w590:string)
            n162 = Decimal String To Number(string=w590, default (0L)=u8 0 ("index (row)")) -> (number=w583:u8)  [unwired: 1 in, 1 out]
            n163 = Replace Array Subset(array=u8[][] [[5, 49, 1, 240, 0, 0, 255]], new element=w583, index (row)=0, index (col)=5 ("disabled index (col)")) -> (w588:u8[][])
            n164 = call "EOL LIN_Send_Single_Message.vi"("NAD"=w584, "Tx Msg"=w588, "LIN Device"=w587) -> ("TxRx Data"=w601:string[][], "Response Good?"=w600:bool, "spreadsheet string"=w586:string, "Rx Msg"=w597:u8[])  [unwired: 8 in, 1 out]
          }
          frame "Hold EOL session" {
            (unwired) u8[][] [[3, 2, 62, 0, 255, 255, 255]]
            n165 = call "EOL LIN_Send_Single_Message.vi"("NAD"=w603, "Tx Msg"=u8[][] [[2, 62, 0, 255, 255, 255, 255]], "LIN Device"=w610) -> ("TxRx Data"=w614:string[][], "Response Good?"=w613:bool, "spreadsheet string"=w606:string, "Rx Msg"=w609:u8[])  [unwired: 8 in, 1 out]
            n166 = call "Elapsed Time2"() -> ("Present (s)"=w607:dbl)  [unwired: 12 in, 7 out]
            n167 = Bundle By Name(cluster=w605, "Hold?"=FALSE ("Hold Mode?"), "Present (s)"=w607) -> (w604:T2)
          }
        }
        n168 = Array To Spreadsheet String(array=w52, 3:"" ("format string")) -> (spreadsheet string=w55:string)  [unwired: 1 in]
        n169 = Concatenate Strings(w51, w55) -> (w53:string)
      }
      frame True {
        n170 = for {
          tunnel: w637 -> [w663]
          tunnel: w636 -> [w662]
          tunnel: [w644] -> w635
          tunnel: [w659] -> w634
          tunnel: [w658] -> w633
          tunnel: [w657] -> w632
          shift-right: [w651] -> w629
          shift-left: w630 -> [w650]
          shift-right: [w660] -> w627
          shift-left: w628 -> [w661]
          tunnel: w626 -> [w649]
          tunnel: w625 -> [w648] mode=indexing
          shift-right: [w656] -> w631
          shift-left: w623 -> [w647]
          tunnel: w622 -> [w646]
          tunnel: w621 -> [w645]
          tunnel: [w643] -> w620
          tunnel: [w642] -> w619
          tunnel: [w641] -> w618
          tunnel: [w640] -> w617
          tunnel: w616 -> [w639]
          tunnel: w615 -> [w638]
          stop <- w644 continue-if-true
          n171 = case shown="\"Enter Diagnostic Mode\"" w648 {
            selector: w648 -> [_ _ _ _ _ _ _ _ _ _ _ _ w986 _ _ _ _ _ _ _ _]
            tunnel: w662 -> [_ w681 w692 w705 w759 w800 w850 w889 w906 w915 w949 w970 w995 w1037 w1133 w1143 w1152 w1165 w1182 w1192 w1215]
            tunnel: [string[][] [] ("TxRx Data") w680 w694 w709 w753 w808 w852 w888 w905 w921 w952 w974 w991 w1042 w1134 w1144 w1156 w1169 w1185 w1206 w1219] -> w652
            tunnel: [TRUE ("Response Good?") w675 w686 w707 w745 w795 w843 w883 w902 w912 w942 w973 w989 w1025 w1128 w1138 w1155 TRUE ("Response Good?") w1176 w1205 w1218] -> w644
            tunnel: w649 -> [_ _ _ _ w741 w791 w838 _ _ w910 w946 w966 w996 w1034 _ _ w1147 w1160 w1173 w1190 _]
            tunnel: w663 -> [_ _ _ _ w751 w789 w848 _ _ w918 w963 w985 w994 w1043 _ _ w1157 w1170 w1186 w1199 _]
            tunnel: ["" ("spreadsheet string") w674 w685 w700 w748 w802 w845 w882 w894 w911 w943 w967 w988 w1024 w1127 w1137 w1148 w1161 w1174 w1191 w1209] -> w659
            tunnel: [u16 0 ("Error No.") u16 9 ("Error No.") u16 178 ("Error No.") w706 u16 68 ("Error No.") u16 62 ("Error No.") u16 69 ("Error No.") u16 181 ("Error No.") w899 u16 82 ("Error No.") u16 184 ("Error No.") u16 185 ("Error No.") u16 20 ("Error No.") u16 20 ("Error No.") u16 55 ("Error No.") u16 55 ("Error No.") u16 56 ("Error No.") u16 0 ("Error No.") u16 56 ("Error No.") u16 186 ("Error No.") u16 187 ("Error No.")] -> w658
            tunnel: [w668 w678 w689 w708 w747 w797 w844 w887 w904 w917 w951 w972 w997 w1039 w1132 w1142 w1154 w1167 w1184 w1204 w1217] -> w656
            tunnel: w647 -> [w668 w678 w688 w708 w747 w797 w844 w887 w904 w917 w951 w972 w997 w1039 w1132 w1142 w1154 w1167 w1184 w1204 w1217]
            tunnel: [u8[] [] ("Rx Message") w677 w689 w704 w743 w793 w840 w885 w896 w914 w948 w969 w992 w1036 w1130 w1140 w1151 w1164 w1180 w1202 w1214] -> w657
            tunnel: w661 -> [w665 w676 w687 w703 w742 w792 w839 w884 w895 w913 w947 w968 w990 w1035 w1129 w1139 w1149 w1162 w1175 w1201 w1211]
            tunnel: [w665 w676 w687 w702 w742 w792 w839 w884 w895 w913 w947 w968 w990 w1035 w1129 w1139 w1149 w1162 w1175 w1201 w1210] -> w660
            tunnel: w646 -> [_ w673 w684 w698 w740 w790 w837 w881 w893 w908 w945 w965 w993 w1033 w1126 w1136 w1146 w1159 w1172 w1189 w1208]
            tunnel: w645 -> [_ _ _ w697 w739 w788 _ _ _ _ w941 _ _ w1023 _ _ _ _ _ _ _]
            tunnel: [_ _ _ _ _ _ w836 _ _ _ _ _ _ _ _ _ _ _ _ _ _] -> w643
            tunnel: [_ _ _ _ _ w787 _ _ _ _ _ _ _ _ _ _ _ _ _ _ _] -> w642
            tunnel: [_ _ _ _ w738 _ _ _ _ _ _ _ _ _ _ _ _ _ _ _ _] -> w641
            tunnel: [_ _ _ _ T1."Softeware version" ("version type") T1."Hardware version" ("version type") T1."Calfile version" ("version type") _ _ _ _ _ _ _ _ _ _ _ _ _ _] -> w640
            tunnel: w639 -> [_ _ _ w696 _ _ _ _ _ _ _ _ _ _ _ _ _ _ _ _ _]
            tunnel: w638 -> [_ _ _ _ _ _ _ _ _ _ w940 _ _ _ _ _ _ _ _ _ _]
            frame Default {
            }
            frame "Enter Diagnostic Mode" {
              (unwired) u8[] [26, 2, 80, 97, 255, 255, 255]
              n172 = call "EOL LIN_Send_Single_Message.vi"("NAD"=w673, "Tx Msg"=u8[][] [[2, 16, 97, 255, 255, 255, 255]], "LIN Device"=w681, "Msg Wait Time"=u32 1000, "Retries"=3) -> ("TxRx Data"=w680:string[][], "Response Good?"=w675:bool, "spreadsheet string"=w674:string, "Rx Msg"=w677:u8[])  [unwired: 6 in, 1 out]
            }
            frame "Request Seed" {
              (unwired) u8[] [26, 4, 103, 97]
              n173 = call "EOL LIN_Send_Single_Message.vi"("NAD"=w684, "Tx Msg"=u8[][] [[2, 39, 97, 255, 255, 255, 255]], "LIN Device"=w692, "Msg Wait Time"=u32 1500) -> ("TxRx Data"=w694:string[][], "Response Good?"=w686:bool, "spreadsheet string"=w685:string, "Rx Msg"=w690:u8[])  [unwired: 7 in, 1 out]
              n174 = Empty Array?(array=w690) -> (empty?=w691:bool)
              n175 = Select(t=w688, s=w691, f=w690) -> (s? t:f=w689:u8[])
            }
            frame "Calculate Key and Send Key" {
              n176 = case shown="\"NU2\", Default" w697 {
                tunnel: [u8[] [4, 39, 2, 255, 255, 255, 255] u8[] [4, 39, 98, 255, 255, 255, 255]] -> w714
                frame "假" {
                }
                frame "NU2", Default {
                }
              }
              n177 = Index Array(array=w708, index #1=4 ("index"), index #2=5 ("index")) -> (element #1=w718:u8, element #2=w717:u8)
              n178 = Join Numbers(hi=w718, lo=w717) -> ((hi.lo)=w712:u16)
              n179 = call "GetKey.vi"("x"=w712) -> ("KEY"=w716:u8[])  [unwired: 10 in]
              n180 = Replace Array Subset(array=w714, new element=w716, index=3) -> (w713:u8[])
              n181 = Equal To 0?(x=w712) -> (x = 0?=w710:bool)
              n182 = Build Array(w713) -> (w711:u8[][])
              n183 = case shown="True" w710 {
                tunnel: w711 -> [w731 _]
                tunnel: [w730 string[][] [] ("TxRx Data")] -> w709
                tunnel: [w729 FALSE ("Response Good?")] -> w707
                tunnel: [w728 w732] -> w700
                tunnel: [u16 180 ("Error No.") u16 179 ("Error No.")] -> w706
                tunnel: w705 -> [w726 _]
                tunnel: [w725 u8[] [] ("Rx Message")] -> w704
                tunnel: w698 -> [w724 _]
                tunnel: w696 -> [_ w732]
                frame False {
                  n184 = call "EOL LIN_Send_Single_Message.vi"("NAD"=w724, "Tx Msg"=w731, "LIN Device"=w726, "Msg Wait Time"=u32 1500) -> ("TxRx Data"=w730:string[][], "Response Good?"=w729:bool, "spreadsheet string"=w728:string, "Rx Msg"=w725:u8[])  [unwired: 7 in, 1 out]
                }
                frame True {
                }
              }
              n185 = call "Elapsed Time3"() -> ("Present (s)"=w701:dbl)  [unwired: 12 in, 7 out]
              n186 = Bundle By Name(cluster=w703, "Hold Mode?"=TRUE, "Present (s)"=w701) -> (w702:T2)
            }
            frame "Check Software Version" {
              n187 = Unflatten From String(type=w751, binary string=w741) -> (value=w752:T5)  [unwired: 3 in, 2 out]
              n188 = case shown="\"假\", Default" w739 {
                tunnel: [u8[][] [[3, 34, 241, 229, 255, 255, 255]] u8[][] [[3, 34, 241, 149, 255, 255, 255]]] -> w760
                frame "假", Default {
                }
                frame "B30", "B41" {
                }
              }
              n189 = Unbundle By Name(w752) -> ("String"=w749:string)
              n190 = call "EOL LIN_Send_Single_Message.vi"("NAD"=w740, "Tx Msg"=w760, "LIN Device"=w759) -> ("TxRx Data"=w753:string[][], "Response Good?"=w746:bool, "Rx Msg"=w743:u8[])  [unwired: 8 in, 2 out]
              n191 = Array Subset(array=w743, index=6, length=2) -> (w758:u8[])
              n192 = for {
                tunnel: w758 -> [w781] mode=indexing
                shift-right: [w784] -> w750
                shift-left: "" -> [w783]
                tunnel: "%02x" ("format string") -> [w782]
                n193 = Format Into String(format string=w782, w781) -> (resulting string=w785:string)  [unwired: 2 in, 1 out]
                n194 = Concatenate Strings(w783, w785) -> (w784:string)
              }
              n195 = case shown="False" w746 {
                tunnel: w750 -> [_ w770]
                tunnel: w749 -> [w764 w769]
                tunnel: [FALSE w772] -> w745
                tunnel: [w763 w768] -> w738
                tunnel: [": Did not get positive response" ("Error Description") w771] -> w748
                frame False {
                  n196 = Build Array("Not read" ("Constant level"), w764) -> (w763:string[])
                }
                frame True {
                  n197 = Equal?(x=w770, y=w769) -> (x = y?=w773:bool)
                  n198 = Concatenate Strings("Actual - " ("string"), w770, ", Set - " ("string"), w769) -> (w774:string)
                  n199 = case shown="True" w773 {
                    tunnel: w774 -> [w777 _]
                    tunnel: [FALSE TRUE] -> w772
                    tunnel: [w777 ""] -> w771
                    frame False {
                    }
                    frame True {
                    }
                  }
                  n200 = Build Array(w770, w769) -> (w768:string[])
                }
              }
            }
            frame "Check Hardware Version" {
              n201 = case shown="\"假\", Default" w788 {
                tunnel: [u8[][] [[3, 34, 241, 227, 255, 255, 255]] u8[][] [[3, 34, 241, 147, 255, 255, 255]]] -> w809
                frame "假", Default {
                }
                frame "B30", "B41" {
                }
              }
              n202 = Unflatten From String(type=w789, binary string=w791) -> (value=w801:T5)  [unwired: 3 in, 2 out]
              n203 = Unbundle By Name(w801) -> ("String"=w799:string)
              n204 = call "EOL LIN_Send_Single_Message.vi"("NAD"=w790, "Tx Msg"=w809, "LIN Device"=w800) -> ("TxRx Data"=w808:string[][], "Response Good?"=w796:bool, "Rx Msg"=w793:u8[])  [unwired: 8 in, 2 out]
              n205 = Array Subset(array=w793, index=6, length=1) -> (w807:u8[])
              n206 = for {
                tunnel: w807 -> [w830] mode=indexing
                shift-right: [w833] -> w798
                shift-left: "" -> [w832]
                tunnel: "%02x" ("format string") -> [w831]
                n207 = Format Into String(format string=w831, w830) -> (resulting string=w834:string)  [unwired: 2 in, 1 out]
                n208 = Concatenate Strings(w832, w834) -> (w833:string)
              }
              n209 = case shown="False" w796 {
                tunnel: w798 -> [_ w819]
                tunnel: w799 -> [w813 w818]
                tunnel: [FALSE w821] -> w795
                tunnel: [w812 w817] -> w787
                tunnel: [": Did not get positive response" ("Error Description") w820] -> w802
                frame False {
                  n210 = Build Array("Not read" ("Constant level"), w813) -> (w812:string[])
                }
                frame True {
                  n211 = Equal?(x=w819, y=w818) -> (x = y?=w822:bool)
                  n212 = Concatenate Strings("Actual - " ("string"), w819, ", Set - " ("string"), w818) -> (w823:string)
                  n213 = case shown="True" w822 {
                    tunnel: w823 -> [w826 _]
                    tunnel: [FALSE TRUE] -> w821
                    tunnel: [w826 ""] -> w820
                    frame False {
                    }
                    frame True {
                    }
                  }
                  n214 = Build Array(w819, w818) -> (w817:string[])
                }
              }
            }
            frame "Check Cal file Version" {
              n215 = Unflatten From String(type=w848, binary string=w838) -> (value=w849:T5)  [unwired: 3 in, 2 out]
              n216 = Unbundle By Name(w849) -> ("String"=w847:string)
              n217 = call "EOL LIN_Send_Single_Message.vi"("NAD"=w837, "Tx Msg"=u8[][] [[3, 34, 252, 1, 255, 255, 255]], "LIN Device"=w850) -> ("TxRx Data"=w852:string[][], "Response Good?"=w842:bool, "Rx Msg"=w840:u8[])  [unwired: 8 in, 2 out]
              n218 = Array Subset(array=w840, index=5, length=2) -> (w857:u8[])
              n219 = for {
                tunnel: w857 -> [w876] mode=indexing
                shift-right: [w879] -> w846
                shift-left: "" -> [w878]
                tunnel: "%02x" ("format string") -> [w877]
                n220 = Format Into String(format string=w877, w876) -> (resulting string=w880:string)  [unwired: 2 in, 1 out]
                n221 = Concatenate Strings(w878, w880) -> (w879:string)
              }
              n222 = case shown="False" w842 {
                tunnel: w846 -> [_ w865]
                tunnel: w847 -> [w859 w864]
                tunnel: [FALSE w867] -> w843
                tunnel: [w858 w863] -> w836
                tunnel: [": Did not get positive response" ("Error Description") w866] -> w845
                frame False {
                  n223 = Build Array("Not read" ("Constant level"), w859) -> (w858:string[])
                }
                frame True {
                  n224 = Equal?(x=w865, y=w864) -> (x = y?=w868:bool)
                  n225 = Concatenate Strings("Actual - " ("string"), w865, ", Set - " ("string"), w864) -> (w869:string)
                  n226 = case shown="True" w868 {
                    tunnel: w869 -> [w872 _]
                    tunnel: [FALSE TRUE] -> w867
                    tunnel: [w872 ""] -> w866
                    frame False {
                    }
                    frame True {
                    }
                  }
                  n227 = Build Array(w865, w864) -> (w863:string[])
                }
              }
            }
            frame "Un-Calibrate SCU" {
              (unwired) u8[] [26, 4, 113, 1, 254, 9]
              n228 = call "EOL LIN_Send_Single_Message.vi"("NAD"=w881, "Tx Msg"=u8[][] [[4, 49, 1, 254, 9, 255, 255]], "LIN Device"=w889) -> ("TxRx Data"=w888:string[][], "Response Good?"=w883:bool, "spreadsheet string"=w882:string, "Rx Msg"=w885:u8[])  [unwired: 8 in, 1 out]
            }
            frame "Check SCU RP and RF status" {
              (unwired) u8[] [26, 5, 98, 253, 254, 9]
              n229 = call "EOL LIN_Send_Single_Message.vi"("NAD"=w893, "Tx Msg"=u8[][] [[3, 34, 253, 1, 255, 255, 255]], "LIN Device"=w906) -> ("TxRx Data"=w905:string[][], "Response Good?"=w903:bool, "spreadsheet string"=w894:string, "Rx Msg"=w896:u8[])  [unwired: 8 in, 1 out]
              n230 = Index Array(array=w896, index=5) -> (element=w892:u8)
              n231 = Equal?(x=w892, y=u8 2 ("element")) -> (x = y?=w891:bool)
              n232 = And(x=w903, y=w891) -> (x .and. y?=w902:bool)
              n233 = Select(t=u16 183 ("Error No."), s=w891, f=u16 182 ("Error No.")) -> (s? t:f=w899:u16)
            }
            frame "Set Cycle Counts" {
              (unwired) u8[] [26, 3, 110, 254, 18]
              n234 = Unflatten From String(type=w918, binary string=w910) -> (value=w938:T5)  [unwired: 3 in, 2 out]
              n235 = Unbundle By Name(w938) -> ("Vent Cycles"=w920:u16, "Slide Cycles"=w919:u16)
              n236 = Split Number(x=w919) -> (hi(x)=w932:u8, lo(x)=w933:u8)
              n237 = Split Number(x=w920) -> (hi(x)=w934:u8, lo(x)=w935:u8)
              n238 = Replace Array Subset(array=u8[] [33, 0, 0, 0, 0, 0, 0] ("Frame payloads to queue"), new element #1=w932, index #1=1 ("索引"), new element #2=w933, index #2=2 ("索引"), new element #3=w934, index #3=3 ("索引"), new element #4=w935, index #4=4 ("索引"), new element #5=w932, index #5=5 ("索引"), new element #6=w933, index #6=6 ("索引")) -> (w937:u8[])
              n239 = Replace Array Subset(array=u8[] [16, 11, 46, 254, 18, 0, 0] ("Frame payloads to queue"), new element #1=w934, index #1=5 ("索引"), new element #2=w935) -> (w936:u8[])  [unwired: 1 in]
              n240 = Build Array(w936, w937) -> (w922:u8[][])
              n241 = call "EOL LIN_Send_Single_Message.vi"("NAD"=w908, "Tx Msg"=w922, "LIN Device"=w915, "Msg Wait Time"=u32 3000) -> ("TxRx Data"=w921:string[][], "Response Good?"=w912:bool, "spreadsheet string"=w911:string, "Rx Msg"=w914:u8[])  [unwired: 7 in, 1 out]
            }
            frame "Go to position glass" {
              n242 = Equal?(x=w941, y=w940) -> (x = y?=w939:bool)
              n243 = Unflatten From String(type=w963, binary string=w946) -> (value=w962:T5)  [unwired: 3 in, 2 out]
              n244 = Unbundle By Name(w962) -> ("Go to Position"=w961:u16)
              n245 = Split Number(x=w961) -> (hi(x)=w958:u8, lo(x)=w957:u8)
              n246 = Replace Array Subset(array=u8[] [33, 0, 0, 0, 0, 255, 255], new element #1=w958, index #1=1 ("index"), new element #2=w957, index #2=2 ("index")) -> (w955:u8[])
              n247 = Build Array(u8[] [16, 9, 49, 1, 253, 4, 1], w955) -> (w953:u8[][])
              n248 = call "EOL LIN_Send_Single_Message.vi"("NAD"=w945, "CD701 position"=w939, "Tx Msg"=w953, "LIN Device"=w949, "Msg Wait Time"=u32 3000) -> ("TxRx Data"=w952:string[][], "Response Good?"=w942:bool, "spreadsheet string"=w943:string, "Rx Msg"=w948:u8[])  [unwired: 6 in, 1 out]
            }
            frame "Go to position sunshade" {
              n249 = Unflatten From String(type=w985, binary string=w966) -> (value=w984:T5)  [unwired: 3 in, 2 out]
              n250 = Unbundle By Name(w984) -> ("Go to Position"=w983:u16)
              n251 = Split Number(x=w983) -> (hi(x)=w980:u8, lo(x)=w979:u8)
              n252 = Replace Array Subset(array=u8[] [33, 0, 0, 0, 0, 255, 255], new element #1=w980, index #1=3 ("index"), new element #2=w979, index #2=4 ("index")) -> (w977:u8[])
              n253 = Build Array(u8[] [16, 9, 49, 1, 253, 4, 2], w977) -> (w975:u8[][])
              n254 = call "EOL LIN_Send_Single_Message.vi"("NAD"=w965, "Tx Msg"=w975, "LIN Device"=w970, "Msg Wait Time"=u32 3000) -> ("TxRx Data"=w974:string[][], "Response Good?"=w973:bool, "spreadsheet string"=w967:string, "Rx Msg"=w969:u8[])  [unwired: 7 in, 1 out]
            }
            frame "Check Cycle Counts" {
              n255 = call "EOL LIN_Send_Single_Message.vi"("NAD"=w993, "Tx Msg"=u8[][] [[3, 34, 254, 18, 255, 255, 255]], "LIN Device"=w995) -> ("TxRx Data"=w991:string[][], "Response Good?"=w1002:bool, "Rx Msg"=w992:u8[])  [unwired: 8 in, 2 out]
              n256 = Unflatten From String(type=w994, binary string=w996) -> (value=w1003:T5)  [unwired: 3 in, 2 out]
              n257 = Index Array(array=w992, index #1=6 ("index")) -> (element #1=w1005:u8, element #2=w1004:u8)  [unwired: 1 in]
              n258 = Unbundle By Name(w1003) -> ("Slide Cycles"=w1000:u16)
              n259 = Join Numbers(hi=w1005, lo=w1004) -> ((hi.lo)=w1001:u16)
              n260 = case shown="True" w1002 {
                tunnel: w1001 -> [_ w1011]
                tunnel: w1000 -> [_ w1010]
                tunnel: ["Could not get reponse during Check Motor Hall Position" ("Error Description") w1012] -> w988
                tunnel: [FALSE w1008] -> w989
                tunnel: w986 -> [_ _]
                frame False {
                }
                frame True {
                  n261 = Equal?(x=w1011, y=w1010) -> (x = y?=w1009:bool)
                  n262 = case shown="True" w1009 {
                    tunnel: [w1016 ""] -> w1012
                    tunnel: w1011 -> [w1015 _]
                    tunnel: w1010 -> [w1014 _]
                    tunnel: [FALSE TRUE] -> w1008
                    frame False {
                      n263 = Format Into String(initial string=", Set - ", w1014) -> (resulting string=w1019:string)  [unwired: 2 in, 1 out]
                      n264 = Format Into String(initial string="Slide Cycle Actual - " ("string"), w1015) -> (resulting string=w1020:string)  [unwired: 2 in, 1 out]
                      n265 = Concatenate Strings(w1020, w1019) -> (w1016:string)
                    }
                    frame True {
                    }
                  }
                }
              }
            }
            frame "Check hall position glass and sunshade" {
              n266 = call "EOL LIN_Send_Single_Message.vi"("NAD"=w1033, "Tx Msg"=u8[][] [[3, 34, 253, 2, 255, 255, 255]], "LIN Device"=w1037) -> ("TxRx Data"=w1042:string[][], "Response Good?"=w1032:bool, "Rx Msg"=w1036:u8[])  [unwired: 8 in, 2 out]
              n267 = Unflatten From String(type=w1043, binary string=w1034) -> (value=w1044:T5)  [unwired: 3 in, 2 out]
              n268 = Index Array(array=w1036, index #1=6 ("index"), index #3=8 ("index")) -> (element #1=w1047:u8, element #2=w1046:u8, element #3=w1041:u8, element #4=w1040:u8)  [unwired: 2 in]
              n269 = Unbundle By Name(w1044) -> ("Check Glass Position"=w1029:u16, "Checkgalss"=w1028:bool, "Check Sunshade Position"=w1027:u16, "Checksunshade"=w1026:bool)
              n270 = Join Numbers(hi=w1047, lo=w1046) -> ((hi.lo)=w1031:u16)
              n271 = Join Numbers(hi=w1041, lo=w1040) -> ((hi.lo)=w1030:u16)
              n272 = case shown="True" w1032 {
                tunnel: w1031 -> [_ w1054]
                tunnel: w1029 -> [_ w1055]
                tunnel: ["Could not get reponse during Check Motor Hall Position" ("Error Description") w1056] -> w1024
                tunnel: [FALSE w1059] -> w1025
                tunnel: w1028 -> [_ w1058]
                tunnel: w1026 -> [_ w1057]
                tunnel: w1030 -> [_ w1053]
                tunnel: w1027 -> [_ w1060]
                tunnel: w1023 -> [_ w1052]
                frame False {
                }
                frame True {
                  n273 = case shown="\"CD701\"" w1052 {
                    tunnel: w1060 -> [_ w1106]
                    tunnel: [w1061 w1103] -> w1059
                    tunnel: w1058 -> [w1062 w1099]
                    tunnel: w1057 -> [_ w1095]
                    tunnel: [w1065 w1091] -> w1056
                    tunnel: w1055 -> [w1063 w1090]
                    tunnel: w1054 -> [w1064 w1086]
                    tunnel: w1053 -> [_ w1085]
                    frame "CD701" {
                      # "只检测玻璃"
                      n274 = Not Equal To 0?(x=w1064) -> (x != 0?=w1075:bool)
                      n275 = Add(x=u16 40, y=w1063) -> (x+y=w1080:u16)
                      n276 = Subtract(x=w1063, y=u16 40) -> (x-y=w1077:u16)
                      n277 = In Range and Coerce(upper limit=w1080, x=w1064, lower limit=w1077) -> (In Range?=w1074:bool)  [unwired: 1 out]
                      n278 = And(x=w1075, y=w1074) -> (x .and. y?=w1073:bool)
                      n279 = Select(t=w1073, s=w1062, f=TRUE) -> (s? t:f=w1061:bool)
                      n280 = Format Into String(initial string=", Max Lt ", w1080) -> (resulting string=w1079:string)  [unwired: 2 in, 1 out]
                      n281 = Format Into String(initial string=", Min Lt ", w1077) -> (resulting string=w1078:string)  [unwired: 2 in, 1 out]
                      n282 = Format Into String(initial string="Glass Actual  " ("string"), w1064) -> (resulting string=w1081:string)  [unwired: 2 in, 1 out]
                      n283 = Concatenate Strings(w1081, w1079, w1078) -> (w1076:string)
                      n284 = Select(t=w1076, s=w1062, f="") -> (s? t:f=w1065:string)
                    }
                    frame "NU2", Default {
                      n285 = Not Equal To 0?(x=w1086) -> (x != 0?=w1089:bool)
                      n286 = Not Equal To 0?(x=w1085) -> (x != 0?=w1084:bool)
                      n287 = Add(x=u16 40, y=w1090) -> (x+y=w1121:u16)
                      n288 = Subtract(x=w1090, y=u16 40) -> (x-y=w1117:u16)
                      n289 = Add(x=u16 20, y=w1106) -> (x+y=w1110:u16)
                      n290 = Subtract(x=w1106, y=u16 20) -> (x-y=w1112:u16)
                      n291 = In Range and Coerce(upper limit=w1121, x=w1086, lower limit=w1117) -> (In Range?=w1088:bool)  [unwired: 1 out]
                      n292 = In Range and Coerce(upper limit=w1110, x=w1085, lower limit=w1112) -> (In Range?=w1083:bool)  [unwired: 1 out]
                      n293 = And(x=w1089, y=w1088) -> (x .and. y?=w1087:bool)
                      n294 = And(x=w1084, y=w1083) -> (x .and. y?=w1082:bool)
                      n295 = Select(t=w1087, s=w1099, f=TRUE) -> (s? t:f=w1105:bool)
                      n296 = Select(t=w1082, s=w1095, f=TRUE) -> (s? t:f=w1104:bool)
                      n297 = And(x=w1105, y=w1104) -> (x .and. y?=w1103:bool)
                      n298 = Format Into String(initial string=", Max Lt ", w1121) -> (resulting string=w1119:string)  [unwired: 2 in, 1 out]
                      n299 = Format Into String(initial string=", Min Lt ", w1117) -> (resulting string=w1118:string)  [unwired: 2 in, 1 out]
                      n300 = Format Into String(initial string="。Sunshade Actual  " ("string"), w1085) -> (resulting string=w1102:string)  [unwired: 2 in, 1 out]
                      n301 = Format Into String(initial string=", Max Lt ", w1110) -> (resulting string=w1101:string)  [unwired: 2 in, 1 out]
                      n302 = Format Into String(initial string=", Min Lt ", w1112) -> (resulting string=w1100:string)  [unwired: 2 in, 1 out]
                      n303 = Format Into String(initial string="Glass Actual  " ("string"), w1086) -> (resulting string=w1125:string)  [unwired: 2 in, 1 out]
                      n304 = Concatenate Strings(w1102, w1101, w1100) -> (w1094:string)
                      n305 = Concatenate Strings(w1125, w1119, w1118) -> (w1098:string)
                      n306 = Select(t=w1098, s=w1099, f="") -> (s? t:f=w1093:string)
                      n307 = Select(t=w1094, s=w1095, f="") -> (s? t:f=w1092:string)
                      n308 = Concatenate Strings(w1093, w1092) -> (w1091:string)
                    }
                  }
                }
              }
            }
            frame "Clear DTC" {
              (unwired) u8[] [26, 1, 84]
              n309 = call "EOL LIN_Send_Single_Message.vi"("NAD"=w1126, "Tx Msg"=u8[][] [[4, 20, 255, 255, 255, 255, 255]], "LIN Device"=w1133) -> ("TxRx Data"=w1134:string[][], "Response Good?"=w1128:bool, "spreadsheet string"=w1127:string, "Rx Msg"=w1130:u8[])  [unwired: 8 in, 1 out]
            }
            frame "Check DTC" {
              (unwired) u8[] [26, 1, 84]
              n310 = call "EOL LIN_Send_Single_Message.vi"("NAD"=w1136, "Tx Msg"=u8[][] [[3, 34, 254, 42, 255, 255, 255]], "LIN Device"=w1143) -> ("TxRx Data"=w1144:string[][], "Response Good?"=w1138:bool, "spreadsheet string"=w1137:string, "Rx Msg"=w1140:u8[])  [unwired: 8 in, 1 out]
            }
            frame "Send Single Message" {
              n311 = Unflatten From String(type=w1157, binary string=w1147) -> (value=w1158:T5)  [unwired: 3 in, 2 out]
              n312 = Unbundle By Name(w1158) -> ("Only Tx1 Bytes"=w1150:u8[][])
              n313 = call "EOL LIN_Send_Single_Message.vi"("NAD"=w1146, "Tx Msg"=w1150, "LIN Device"=w1152) -> ("TxRx Data"=w1156:string[][], "Response Good?"=w1155:bool, "spreadsheet string"=w1148:string, "Rx Msg"=w1151:u8[])  [unwired: 8 in, 1 out]
            }
            frame "Send Single Message With Out Rx" {
              n314 = Unflatten From String(type=w1170, binary string=w1160) -> (value=w1171:T5)  [unwired: 3 in, 2 out]
              n315 = Unbundle By Name(w1171) -> ("Only Tx1 Bytes"=w1163:u8[][])
              n316 = call "EOL LIN_Send_Single_Message.vi"("NAD"=w1159, "Tx Msg"=w1163, "LIN Device"=w1165) -> ("TxRx Data"=w1169:string[][], "spreadsheet string"=w1161:string, "Rx Msg"=w1164:u8[])  [unwired: 8 in, 2 out]
            }
            frame "Send Single Message With Response" {
              n317 = Unflatten From String(type=w1186, binary string=w1173) -> (value=w1187:T5)  [unwired: 3 in, 2 out]
              n318 = Unbundle By Name(w1187) -> ("Tx Bytes"=w1181:u8[][], "Rx Bytes"=w1179:u8[])
              n319 = call "EOL LIN_Send_Single_Message.vi"("NAD"=w1172, "Tx Msg"=w1181, "LIN Device"=w1182) -> ("TxRx Data"=w1185:string[][], "Response Good?"=w1178:bool, "spreadsheet string"=w1174:string, "Rx Msg"=w1180:u8[])  [unwired: 8 in, 1 out]
              n320 = call "Check Response Bytes.vi"("Data Bytes"=w1179, "Response Bytes"=w1180) -> ("Pass?"=w1177:bool)  [unwired: 9 in]
              n321 = And(x=w1178, y=w1177) -> (x .and. y?=w1176:bool)
            }
            frame "Inalfa SCU Teach" {
              n322 = Unflatten From String(type=w1199, binary string=w1190) -> (value=w1200:T5)  [unwired: 3 in, 2 out]
              n323 = Unbundle By Name(w1200) -> ("String"=w1195:string)
              n324 = Decimal String To Number(string=w1195, default (0L)=u8 0 ("index (row)")) -> (number=w1188:u8)  [unwired: 1 in, 1 out]
              n325 = Replace Array Subset(array=u8[][] [[5, 49, 1, 240, 0, 0, 255]], new element=w1188, index (row)=0, index (col)=5 ("disabled index (col)")) -> (w1193:u8[][])
              n326 = call "EOL LIN_Send_Single_Message.vi"("NAD"=w1189, "Tx Msg"=w1193, "LIN Device"=w1192) -> ("TxRx Data"=w1206:string[][], "Response Good?"=w1205:bool, "spreadsheet string"=w1191:string, "Rx Msg"=w1202:u8[])  [unwired: 8 in, 1 out]
            }
            frame "Hold EOL session" {
              (unwired) u8[][] [[3, 2, 62, 0, 255, 255, 255]]
              n327 = call "EOL LIN_Send_Single_Message.vi"("NAD"=w1208, "Tx Msg"=u8[][] [[2, 62, 0, 255, 255, 255, 255]], "LIN Device"=w1215) -> ("TxRx Data"=w1219:string[][], "Response Good?"=w1218:bool, "spreadsheet string"=w1209:string, "Rx Msg"=w1214:u8[])  [unwired: 8 in, 1 out]
              n328 = call "Elapsed Time4"() -> ("Present (s)"=w1212:dbl)  [unwired: 12 in, 7 out]
              n329 = Bundle By Name(cluster=w1211, "Hold?"=FALSE ("Hold Mode?"), "Present (s)"=w1212) -> (w1210:T2)
            }
          }
          n330 = Array To Spreadsheet String(array=w652, 3:"" ("format string")) -> (spreadsheet string=w654:string)  [unwired: 1 in]
          n331 = Wait (ms)(milliseconds to wait=u32 20) -> ()  [unwired: 1 out]
          n332 = Concatenate Strings(w650, w654) -> (w651:string)
        }
      }
    }
    "Error Description" <- w35
    "Error No." <- w26
    "Rx Message" <- w20
    "data bytes log out" <- w23
    "Software version" <- w9
    "Hardware version" <- w8
    "Calfile version" <- w7
    "version type" <- w6
    n333 = Not(x=w3) -> (.not. x?=w4:bool)
    n334 = And(x=w19, y=w4) -> (x .and. y?=w18:bool)
    n335 = case shown="False" w18 {
      selector: w18 -> [w1220 w1225]
      tunnel: w21 -> [w1222 w1228]
      tunnel: [w1221 w1227] -> w28
      tunnel: w3 -> [w1223 _]
      tunnel: [w1223 TRUE ("Response Good?")] -> w27
      frame False {
        n336 = Bundle By Name(cluster=w1222, "Rx Invalid?"=w1220) -> (w1221:T2)
      }
      frame True {
        n337 = Bundle By Name(cluster=w1228, "Hold Mode?"=FALSE, "Rx Invalid?"=w1225) -> (w1227:T2)
      }
    }
    "Response Good?" <- w27
    "Sequence State out" <- w28
    n338 = Wait (ms)(milliseconds to wait=u32 20) -> ()  [unwired: 1 out]
  }
